vi "Generate JSON Report.vi"() -> ()   [LabVIEW 2014, in "i3-docs.lvlib"]
uses:
  i3-docs.lvlib
  Controls/config_fgv_actions.ctl
  Controls/config.ctl
  Controls/current_config.ctl
panel:
  out "Projects Progress":enum32{"Multiple Projects", "Single Project"}(tab)
  out "Projects Completed (%)":dbl(slide) scale=0.0..100.0
  out "Current Output Directory":path
  out "Current Project File":path
  out "Total Project Items Processed":i32 caption="Total Project Items Processed (May be different from final counts due to skipped types, errors, etc)"
  out "Running Time (s)":dbl
  out "Current Project Item":string
  # "Note: Total Project Items Processed may be different from final counts due because it includes skipped types, errors, etc"
  # "Just one project to execute"
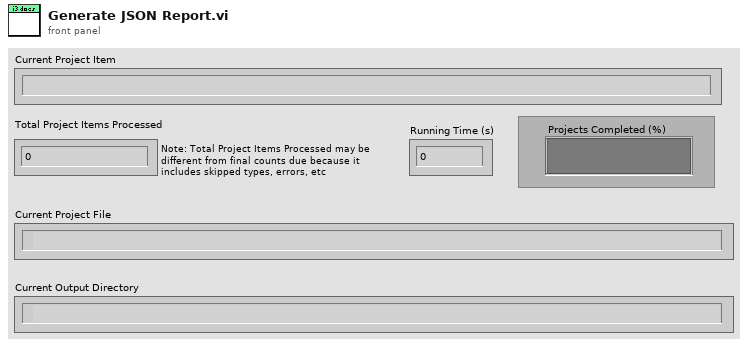
[diagram p1: front panel]
types:
  T1 = typedef "i3-docs.lvlib/config_fgv_actions.ctl" = enum16{"Initialize", "Set Current Project", "Get Current Config", "Set Current Project Item", "Finished"}
  T2 = typedef "i3-docs.lvlib/config.ctl" = cluster{"Current Project":i32, "Project Configurations":T3[], "Current Project Item":string, "Finished?":bool, "Total Project Items":i32, "Disable Delete Output Directories Warning?":bool}
  T3 = typedef "i3-docs.lvlib/current_config.ctl" = cluster{"project file":path, "output directory":path}
  T4 = enum16{"open", "replace", "create", "open or create", "replace or create", "replace or create with confirmation"}
  T5 = typedef "i3-docs.lvlib/project_item.ctl" = cluster{"type":string, "owned_items":string[], "item_id":string, "display_name":string, "description":string, "block_diagram_images":T6[], "icon_image":T6}
  T6 = typedef "i3-docs.lvlib/image_information.ctl" = cluster{"file_name":string, "height":i32, "width":i32}
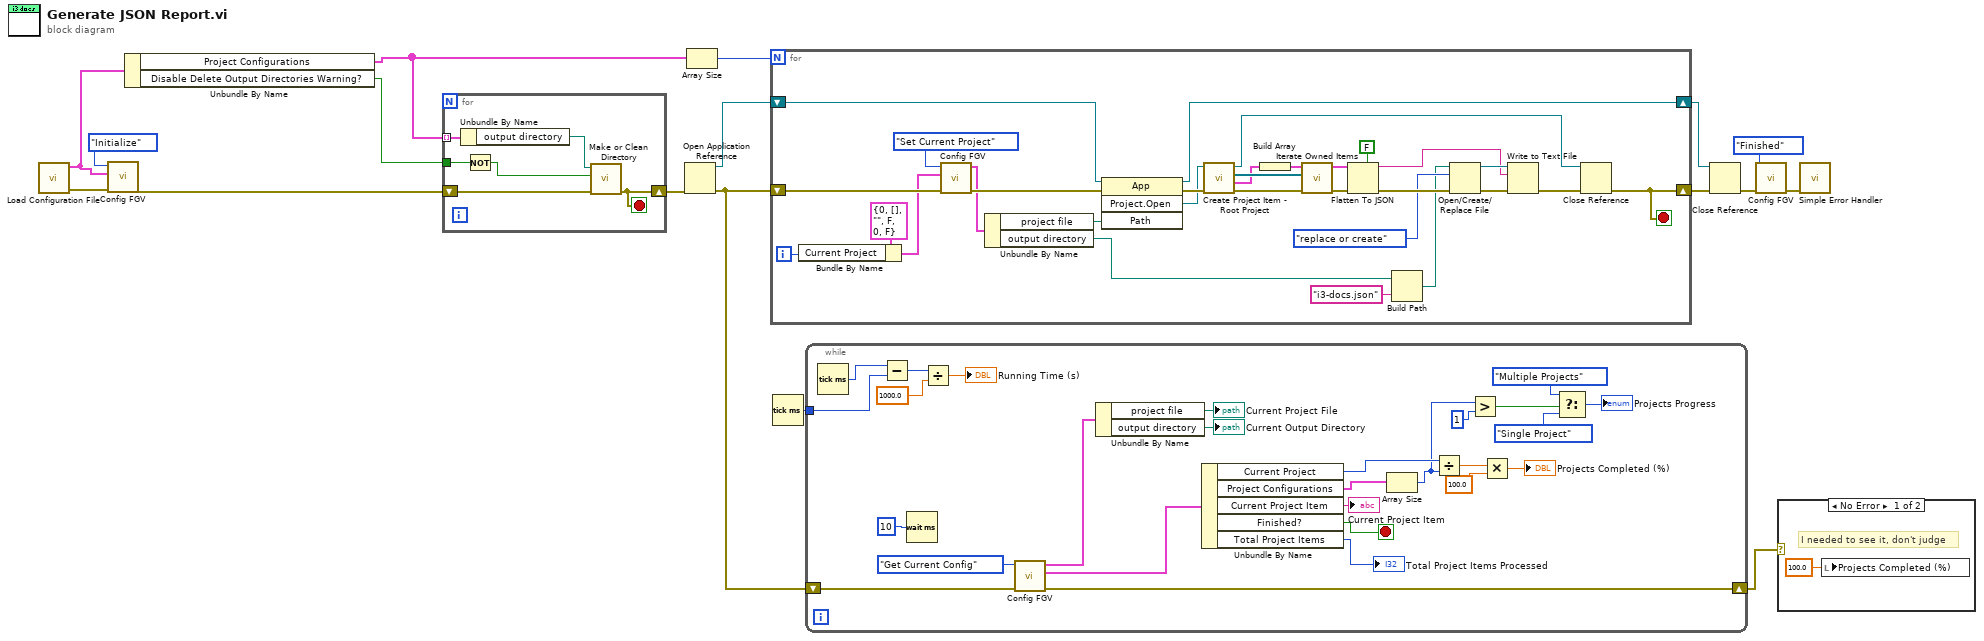
[diagram p0: block diagram]
diagram:
  n1 = call "Load Configuration File.vi"() -> ("Error Out"=w15:errorcluster, "Application Configuration"=w14:T2)  [unwired: 10 in]
  n2 = call "Config FGV.vi"("Error In"=w15, "Application Configuration Input Helper"=w14, "Action"=config_fgv_actions."Initialize") -> ("Error Out"=w2:errorcluster)  [unwired: 6 in, 2 out]
  n3 = Unbundle By Name(w14) -> ("Project Configurations"=w4:T3[], "Disable Delete Output Directories Warning?"=w1:bool)
  n4 = for {
    tunnel: w4 -> [w23] mode=indexing
    shift-right: [w21] -> w3
    shift-left: w2 -> [w22]
    tunnel: w1 -> [w19]
    stop <- w21 stop-if-true
    n5 = Unbundle By Name(w23) -> ("output directory"=w20:path)
    n6 = Not(x=w19) -> (.not. x?=w18:bool)
    n7 = call "Make or Clean Directory.vi"("Error In"=w22, "Warn before delete? (T)"=w18, "File Path to Make or Clean"=w20) -> ("Error Out"=w21:errorcluster)  [unwired: 7 in, 1 out]
  }
  n8 = Open Application Reference(8:w3) -> (0:w6:errorcluster, 3:w17:refnum<vi>)  [unwired: 3 in]
  n9 = Array Size(array=w4) -> (size(s)=w13:i32)
  n10 = for {
    N: w13 -> [_]
    shift-right: [w28] -> w12
    shift-left: w6 -> [w40]
    shift-right: [w30] -> w11
    shift-left: w17 -> [w31]
    i -> [w25]
    stop <- w28 stop-if-true
    n11 = Bundle By Name(cluster=T2 {"Current Project"=0, "Project Configurations"=[], "Current Project Item"="", "Finished?"=FALSE, "Total Project Items"=0, "Disable Delete Output Directories Warning?"=FALSE} ("Config Helper"), "Current Project"=w25) -> (w24:T2)
    n12 = call "Config FGV.vi"("Error In"=w40, "Application Configuration Input Helper"=w24, "Action"=config_fgv_actions."Set Current Project") -> ("Error Out"=w39:errorcluster, "Current Project Configuration"=w36:T3)  [unwired: 6 in, 1 out]
    n13 = Unbundle By Name(w36) -> ("project file"=w34:path, "output directory"=w33:path)
    n14 = invoke class="App" method="Project.Open"(reference=w31, error in=w39, "Path"=w34) -> (reference out=w30:refnum<vi>, error out=w38:errorcluster, "Project:Open"=w37:refnum<vi>)  [unwired: 1 in, 1 out]
    n15 = call "Create Project Item - Root Project.vi"("Error In"=w38, "Project Reference"=w37) -> ("Error Out"=w44:errorcluster, "project item"=w41:T5, "Owned Items[]"=w43:refnum<vi>[], "Project Reference Out"=w27:refnum<vi>)  [unwired: 6 in]
    n16 = Build Array(w41) -> (w42:T5[])
    n17 = call "Iterate Owned Items.vi"("Error In"=w44, "Owned Items[]"=w43, "Project Items In"=w42) -> ("Error Out"=w46:errorcluster, "Project Items Out"=w45:T5[])  [unwired: 7 in]
    n18 = Flatten To JSON(enable LabVIEW extensions? (T)=FALSE, anything=w45, error in (no error)=w46) -> (JSON string=w47:string, 11:w53:errorcluster)
    n19 = Build Path(base path=w33, name or relative path="i3-docs.json") -> (appended path=w49:path)
    n20 = Open/Create/Replace File(file path (use dialog)=w49, error in=w53, operation (0:open)=T4."replace or create") -> (refnum out=w48:refnum<file>, error out=w51:errorcluster)  [unwired: 3 in, 1 out]
    n21 = Write to Text File(file (use dialog)=w48, text=w47, error in=w51) -> (error out=w29:errorcluster)  [unwired: 1 in, 2 out]
    n22 = Close Reference(reference=w27, error in (no error)=w29) -> (error out=w28:errorcluster)
  }
  n23 = Tick Count (ms)() -> (millisecond timer value=w7:u32)
  n24 = while {
    tunnel: w7 -> [w74]
    shift-right: [w69] -> w5
    shift-left: w6 -> [w70]
    stop <- w77 stop-if-true
    n25 = Tick Count (ms)() -> (millisecond timer value=w75:u32)
    n26 = Subtract(x=w75, y=w74) -> (x-y=w73:u32)
    n27 = Wait (ms)(milliseconds to wait=u32 10) -> ()  [unwired: 1 out]
    n28 = Divide(x=w73, y=1000.0) -> (x/y=→"Running Time (s)":dbl)
    n29 = call "Config FGV.vi"("Error In"=w70, "Action"=config_fgv_actions."Get Current Config") -> ("Error Out"=w69:errorcluster, "Full Application Configuration"=w78:T2, "Current Project Configuration"=w67:T3)  [unwired: 7 in]
    n30 = Unbundle By Name(w67) -> ("project file"=→"Current Project File":path, "output directory"=→"Current Output Directory":path)
    n31 = Unbundle By Name(w78) -> ("Current Project"=w63:i32, "Project Configurations"=w64:T3[], "Current Project Item"=→"Current Project Item":string, "Finished?"=w77:bool, "Total Project Items"=→"Total Project Items Processed":i32)
    n32 = Array Size(array=w64) -> (size(s)=w56:i32)
    n33 = Divide(x=w63, y=w56) -> (x/y=w62:dbl)
    n34 = Greater?(x=w56, y=1) -> (0:w54:bool)
    n35 = Multiply(x=w62, y=100.0) -> (x*y=→"Projects Completed (%)":dbl)
    n36 = Select(t=enum32{"Multiple Projects", "Single Project"}."Multiple Projects" ("Tab Control"), s=w54, f=enum32{"Multiple Projects", "Single Project"}."Single Project" ("Tab Control")) -> (s? t:f=→"Projects Progress":enum32{"Multiple Projects", "Single Project"})
  }
  n37 = Close Reference(reference=w11, error in (no error)=w12) -> (error out=w10:errorcluster)
  n38 = call "Config FGV.vi"("Error In"=w10, "Action"=config_fgv_actions."Finished") -> ("Error Out"=w9:errorcluster)  [unwired: 7 in, 2 out]
  n39 = case shown="No Error" w5 {
    frame No Error {
      # "I needed to see it, don't judge"
      n40 = local write "Projects Completed (%)"(100.0 ("Projects Completed (%)")) -> ()
    }
    frame Error {
    }
  }
  n41 = call <vilib>:"Simple Error Handler.vi"("error in (no error)"=w9) -> ()  [unwired: 4 in, 5 out]
